vi "RectPoly.vi"(10 "Height":dbl, 11 "Width":dbl) -> (3 "VertexArray":T1[](array[typedef]))   [LabVIEW 2014]
uses:
  TypeDefs/Point2DwSlope.ctl
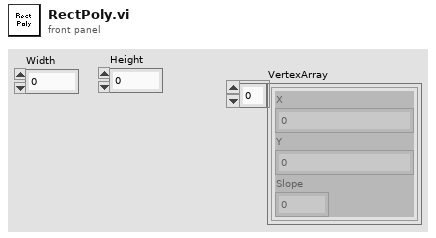
[diagram p1: front panel]
types:
  T1 = typedef "Point2DwSlope.ctl" = cluster{"X":sgl, "Y":sgl, "Slope":dbl}
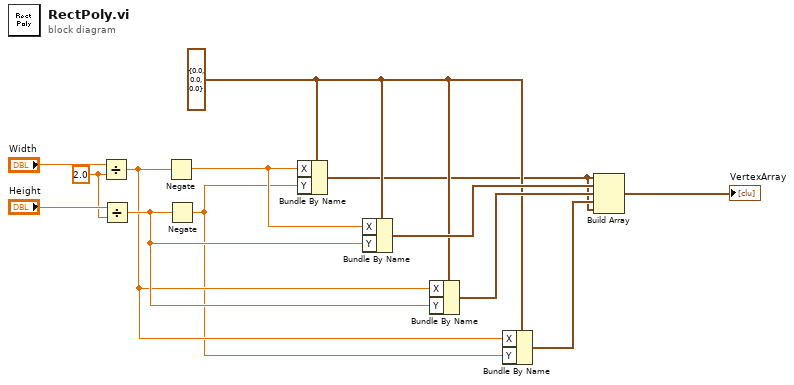
[diagram p0: block diagram]
diagram:
  w3 = T1 {"X"=0.0, "Y"=0.0, "Slope"=0.0} ("Point2D")
  w11 = 2.0 ("y")
  n1 = Divide(x="Width", y=w11) -> (x/y=w8:dbl)
  n2 = Divide(x="Height", y=w11) -> (x/y=w9:dbl)
  n3 = Negate(x=w8) -> (-x=w10:dbl)
  n4 = Negate(x=w9) -> (-x=w7:dbl)
  n5 = Bundle By Name(cluster=w3, "X"=w10, "Y"=w7) -> (w1:T1)
  n6 = Bundle By Name(cluster=w3, "X"=w10, "Y"=w9) -> (w6:T1)
  n7 = Bundle By Name(cluster=w3, "X"=w8, "Y"=w9) -> (w5:T1)
  n8 = Bundle By Name(cluster=w3, "X"=w8, "Y"=w7) -> (w4:T1)
  n9 = Build Array(w1, w6, w5, w4, w1) -> (→"VertexArray":T1[])
